vi "Reference pressure module - Configure.vi"() -> ()   [LabVIEW 2020]
uses:
  Arduino/ctls_and_globals/Arduino tx msg cluster.ctl
panel:
  in  "N averaging":u32=300
  in  "Baud rate (bps)":u32=476000
  in  "Address":u8=1
  in  "Port":refnum<visa-resource-name>
  in  "Get / Set":u8(ring) items=["Get", "Set"]
  out "Read-back":string
  out "Status comment":string
  in  "Address":u8=1
  # "Use this vi to configure the tunnel reference pressure transducer nodes\nThese settings are retained in EEPROM and recalled on power-up."
  # "PN 23/07/2023"
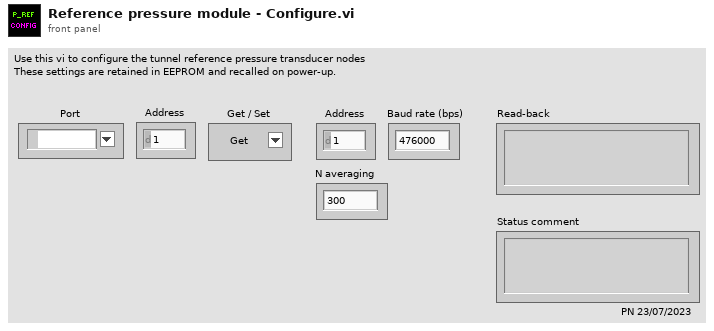
[diagram p1: front panel]
types:
  T1 = typedef "Arduino tx msg cluster.ctl" = cluster{"dest":u8, "A/D/C/I":string, "R/W":string, "chan":u8, "val (float)":sgl}
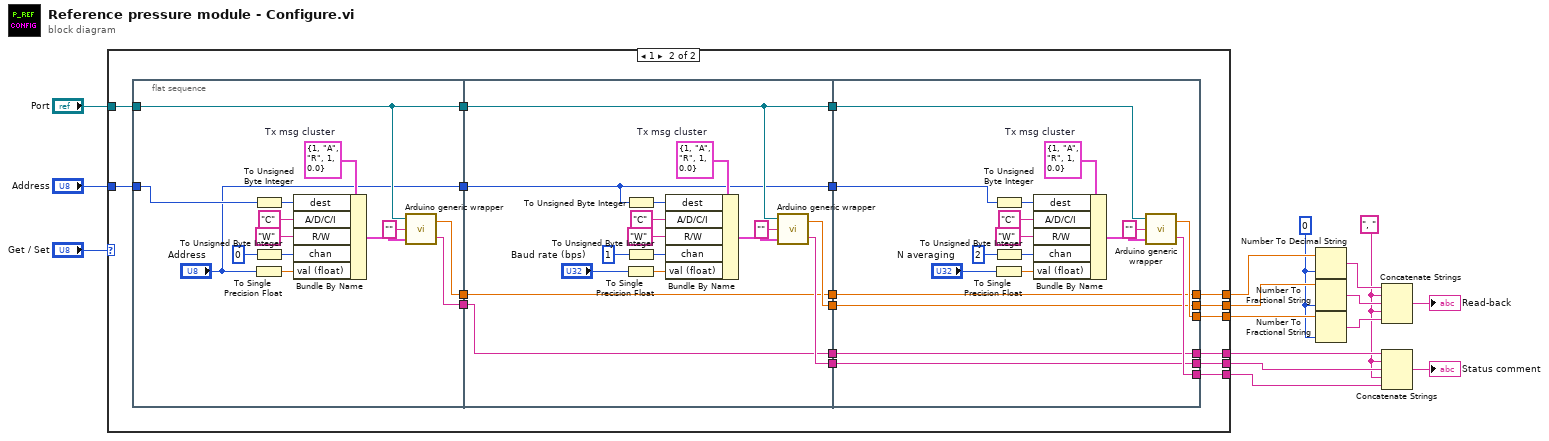
[diagram p0: block diagram]
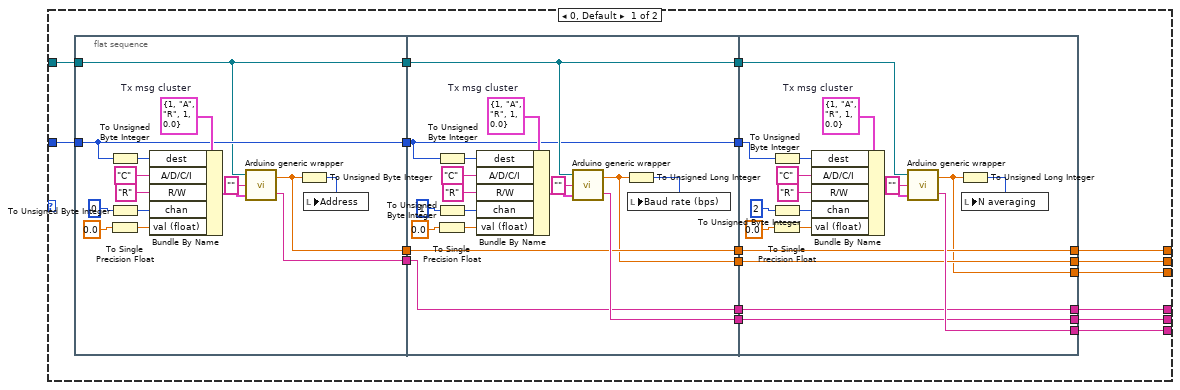
[diagram p2: hidden frame]
diagram:
  w2 = i16 0 ("precision (6)")
  w1 = ", "
  n1 = case shown="1" "Get / Set" {
    tunnel: "Address" -> [w23 w93]
    tunnel: [w20 w92] -> w11
    tunnel: [w17 w91] -> w10
    tunnel: [w18 w90] -> w9
    tunnel: [w19 w89] -> w8
    tunnel: [w21 w88] -> w7
    tunnel: [w22 w86] -> w6
    tunnel: "Port" -> [w24 w87]
    frame 0, Default {
      n2 = flat-sequence {
        tunnel: w23 -> [w41]
        tunnel: w24 -> [w40]
        tunnel: [w40] -> w34
        tunnel: [w41] -> w33
        tunnel: [w36] -> w32
        tunnel: [w39] -> w31
        tunnel: [w58] -> w30
        tunnel: [w57] -> w29
        tunnel: [w56] -> w28
        tunnel: [w51] -> w27
        tunnel: w34 -> [w58]
        tunnel: w33 -> [w57]
        tunnel: w32 -> [w54]
        tunnel: w31 -> [w55]
        tunnel: [w55] -> w26
        tunnel: [w54] -> w25
        tunnel: w30 -> [w77]
        tunnel: w29 -> [w76]
        tunnel: w28 -> [w74]
        tunnel: w27 -> [w72]
        tunnel: w26 -> [w73]
        tunnel: w25 -> [w71]
        tunnel: [w68] -> w20
        tunnel: [w75] -> w17
        tunnel: [w74] -> w18
        tunnel: [w73] -> w19
        tunnel: [w72] -> w21
        tunnel: [w71] -> w22
        frame #0 {
          w49 = T1 {"dest"=1, "A/D/C/I"="A", "R/W"="R", "chan"=1, "val (float)"=0.0}  # Tx msg cluster
          n3 = To Unsigned Byte Integer(number=w41) -> (unsigned 8bit integer=w47:u8)
          n4 = To Unsigned Byte Integer(number=u8 0) -> (unsigned 8bit integer=w48:u8)
          n5 = To Single Precision Float(number=0.0) -> (single precision float=w45:sgl)
          n6 = Bundle By Name(cluster=w49, "dest"=w47, "A/D/C/I"="C" ("A/D"), "R/W"="R", "chan"=w48, "val (float)"=w45) -> (w46:T1)
          n7 = call "Arduino generic wrapper.vi"("Tx msg cluster"=w46, "Channel Name"="", "Port name"=w40) -> ("Scan comment"=w39:string, "Output"=w36:dbl)
          n8 = To Unsigned Byte Integer(number=w36) -> (unsigned 8bit integer=w35:u8)
          n9 = local write "Address"(w35) -> ()
        }
        frame #1 {
          w59 = T1 {"dest"=1, "A/D/C/I"="A", "R/W"="R", "chan"=1, "val (float)"=0.0}  # Tx msg cluster
          n10 = To Unsigned Byte Integer(number=w57) -> (unsigned 8bit integer=w61:u8)
          n11 = To Unsigned Byte Integer(number=u8 1) -> (unsigned 8bit integer=w60:u8)
          n12 = To Single Precision Float(number=0.0) -> (single precision float=w63:sgl)
          n13 = Bundle By Name(cluster=w59, "dest"=w61, "A/D/C/I"="C" ("A/D"), "R/W"="R", "chan"=w60, "val (float)"=w63) -> (w62:T1)
          n14 = call "Arduino generic wrapper.vi"("Tx msg cluster"=w62, "Channel Name"="", "Port name"=w58) -> ("Scan comment"=w56:string, "Output"=w51:dbl)
          n15 = To Unsigned Long Integer(number=w51) -> (unsigned 32bit integer=w50:u32)
          n16 = local write "Baud rate (bps)"(w50) -> ()
        }
        frame #2 {
          w85 = T1 {"dest"=1, "A/D/C/I"="A", "R/W"="R", "chan"=1, "val (float)"=0.0}  # Tx msg cluster
          n17 = To Unsigned Byte Integer(number=w76) -> (unsigned 8bit integer=w83:u8)
          n18 = To Unsigned Byte Integer(number=u8 2) -> (unsigned 8bit integer=w84:u8)
          n19 = To Single Precision Float(number=0.0) -> (single precision float=w81:sgl)
          n20 = Bundle By Name(cluster=w85, "dest"=w83, "A/D/C/I"="C" ("A/D"), "R/W"="R", "chan"=w84, "val (float)"=w81) -> (w82:T1)
          n21 = call "Arduino generic wrapper.vi"("Tx msg cluster"=w82, "Channel Name"="", "Port name"=w77) -> ("Scan comment"=w75:string, "Output"=w68:dbl)
          n22 = To Unsigned Long Integer(number=w68) -> (unsigned 32bit integer=w67:u32)
          n23 = local write "N averaging"(w67) -> ()
        }
      }
    }
    frame 1 {
      n24 = flat-sequence {
        tunnel: w93 -> [w109]
        tunnel: w87 -> [w108]
        tunnel: [w108] -> w103
        tunnel: ["Address"] -> w102
        tunnel: [w107] -> w101
        tunnel: [w106] -> w100
        tunnel: [w125] -> w99
        tunnel: [w124] -> w98
        tunnel: [w123] -> w97
        tunnel: [w122] -> w96
        tunnel: w103 -> [w125]
        tunnel: w102 -> [w124]
        tunnel: w101 -> [w120]
        tunnel: w100 -> [w121]
        tunnel: [w121] -> w95
        tunnel: [w120] -> w94
        tunnel: w99 -> [w143]
        tunnel: w98 -> [w142]
        tunnel: w97 -> [w139]
        tunnel: w96 -> [w137]
        tunnel: w95 -> [w138]
        tunnel: w94 -> [w134]
        tunnel: [w140] -> w92
        tunnel: [w141] -> w91
        tunnel: [w139] -> w90
        tunnel: [w138] -> w89
        tunnel: [w137] -> w88
        tunnel: [w134] -> w86
        frame #0 {
          w117 = T1 {"dest"=1, "A/D/C/I"="A", "R/W"="R", "chan"=1, "val (float)"=0.0}  # Tx msg cluster
          n25 = To Unsigned Byte Integer(number=w109) -> (unsigned 8bit integer=w115:u8)
          n26 = To Unsigned Byte Integer(number=u8 0) -> (unsigned 8bit integer=w116:u8)
          n27 = To Single Precision Float(number="Address") -> (single precision float=w113:sgl)
          n28 = Bundle By Name(cluster=w117, "dest"=w115, "A/D/C/I"="C" ("A/D"), "R/W"="W", "chan"=w116, "val (float)"=w113) -> (w114:T1)
          n29 = call "Arduino generic wrapper.vi"("Tx msg cluster"=w114, "Channel Name"="", "Port name"=w108) -> ("Scan comment"=w106:string, "Output"=w107:dbl)
        }
        frame #1 {
          w126 = T1 {"dest"=1, "A/D/C/I"="A", "R/W"="R", "chan"=1, "val (float)"=0.0}  # Tx msg cluster
          n30 = To Unsigned Byte Integer(number=w124) -> (unsigned 8bit integer=w128:u8)
          n31 = To Unsigned Byte Integer(number=u8 1) -> (unsigned 8bit integer=w127:u8)
          n32 = To Single Precision Float(number="Baud rate (bps)") -> (single precision float=w130:sgl)
          n33 = Bundle By Name(cluster=w126, "dest"=w128, "A/D/C/I"="C" ("A/D"), "R/W"="W", "chan"=w127, "val (float)"=w130) -> (w129:T1)
          n34 = call "Arduino generic wrapper.vi"("Tx msg cluster"=w129, "Channel Name"="", "Port name"=w125) -> ("Scan comment"=w123:string, "Output"=w122:dbl)
        }
        frame #2 {
          w151 = T1 {"dest"=1, "A/D/C/I"="A", "R/W"="R", "chan"=1, "val (float)"=0.0}  # Tx msg cluster
          n35 = To Unsigned Byte Integer(number=w142) -> (unsigned 8bit integer=w149:u8)
          n36 = To Unsigned Byte Integer(number=u8 2) -> (unsigned 8bit integer=w150:u8)
          n37 = To Single Precision Float(number="N averaging") -> (single precision float=w147:sgl)
          n38 = Bundle By Name(cluster=w151, "dest"=w149, "A/D/C/I"="C" ("A/D"), "R/W"="W", "chan"=w150, "val (float)"=w147) -> (w148:T1)
          n39 = call "Arduino generic wrapper.vi"("Tx msg cluster"=w148, "Channel Name"="", "Port name"=w143) -> ("Scan comment"=w141:string, "Output"=w140:dbl)
        }
      }
    }
  }
  n40 = Number To Decimal String(number=w6, width (-)=w2) -> (decimal integer string=w15:string)
  n41 = Number To Fractional String(number=w7, precision (6)=w2) -> (F-format string=w14:string)  [unwired: 2 in]
  n42 = Number To Fractional String(number=w11, precision (6)=w2) -> (F-format string=w5:string)  [unwired: 2 in]
  n43 = Concatenate Strings(w15, w1, w14, w1, w5) -> (→"Read-back":string)
  n44 = Concatenate Strings(w8, w1, w9, w1, w10) -> (→"Status comment":string)
